vi "Wind_Turbine.vi"() -> (5 "Plug in titles":string[](array[string]), 7 "Plug in values":string[](array[string]))   [LabVIEW 2012]
uses:
  Globals/Meas_global.vi
  Globals/LDA_meas_global_1.vi
  <vilib>/Analysis/baseanly.llb/Mean (DBL).vi
  <vilib>/Analysis/NI_AALBase.lvlib
  <vilib>/Analysis/NI_AALPro.lvlib
panel:
  out "Blade 3 Every Pass":dbl[](graph)
  out "Blade 2 Every Pass":dbl[](graph)
  out "Blade 1 Every Pass":dbl[](graph)
  out "Blade Angles":dbl[][](graph)
  out "Blade Analysis":string[][](table)
  out "Blade Positions":dbl[][](graph)
  in  "Allow large changes?":bool
  out "Turbine RPMs":cluster{i32[], "All WTs":dbl[]}(graph)
  out "WT Numbers":string[](array[string])
  out "XY Graph":cluster{dbl[], dbl[]}[](graph)
  out "WT Revolution Start times":dbl[](array[numeric])
  out "Angle 3":dbl format="%#_3g"
  out "Angle 2":dbl format="%#_3g"
  out "Angle 1":dbl format="%#_3g"
  out "L Status Phase lock index":i32
  out "Laser Status Index":i32
  out "Laser Phase lock index":i32
  out "Laser Disp Index":i32
  out "Av Variance 3":dbl
  out "Av Variance 2":dbl
  out "Av Variance 1":dbl
  out "slope 3":dbl format="%#_3g"
  out "slope 2":dbl format="%#_3g"
  out "Mean Blade 3":cluster{dbl, "Angular Step":dbl, dbl[]}(graph)
  out "Mean Blade 2":cluster{dbl, "Angular Step":dbl, dbl[]}(graph)
  out "Av Disp 3":dbl
  out "Av Disp 2":dbl
  out "Av Disp 1":dbl
  out "slope 1":dbl format="%#_3g"
  in  "End Cut Deg":dbl
  in  "Start Cut Deg":dbl
  out "Mean Blade 1":cluster{dbl, "Angular Step":dbl, dbl[]}(graph)
  in  "Angular Step":dbl=1.0
  in  "Turbine to Phase Lock to":u16(ring) items=["RV (WT1)"]
  in  "Change Dem Voltages?":bool=TRUE
  out "All WTs":dbl[][](array[numeric]) format="%#.2g"
  out "WT trace index":dbl[][](array[numeric])
  in  "precision":string
  in  "Add Phase data to results file":bool
  in  "Separation Character":string="\t"
  in  "Output Directory":path
  in  "Save Phase averaged Profiles":bool
  out "Pulses per Rev":i32
  in  "Channel to Phase lock":i32[](listbox)
  # "Mean RPM      SD RPM           Max-Min"
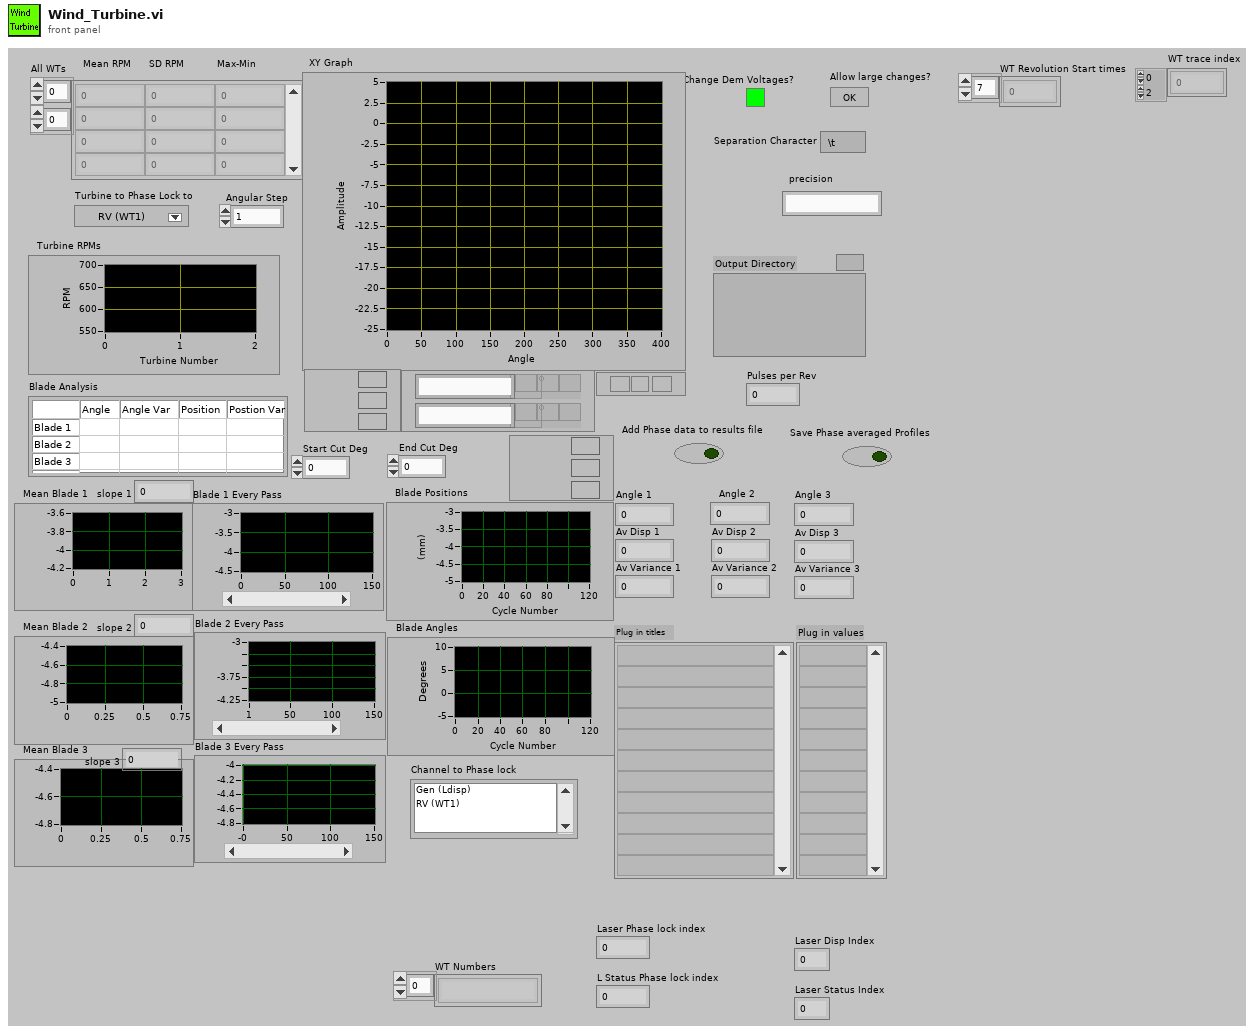
[diagram p1: front panel]
types:
  T1 = typedef "Post_Process.ctl" = enum16{"Take New Data", "Post Process Raw Data File"}
  T2 = typedef "Analysis_info_cluster.ctl" = cluster{"Colour":u32, "Inst type":T3, "Inst name":string, "Symbol":string, "Code name":string, "Extra Info":string, "Inst Array":T4, "Extra Titles":string[], "Extra Values":string[], "U":dbl, "u^2":dbl, "u^3":dbl, "u^4":dbl, "Skew_u":dbl, "Kurt_u":dbl, "Sd Error in Mean":dbl, "% u'/U":dbl, "X":dbl, "Y":dbl, "Z":dbl, "Timescale integral to 25%":dbl, "Sd Error in Variance":dbl, "Calib File":path, "Calib Constants":dbl[], "Output Position":bool, "Full Stats":bool, "Av Sampling Rate":dbl, "Av No of Samples":dbl, "Total Meas Time (s)":dbl, "ADAM Ch Name":string}
  T3 = typedef "Inst_type.ctl" = enum16{"Propeller anemometer", "Raw voltage", "Pressure Transducer", "Pitot-static tube", "Preston tube", "Hot wire", "Cross wire 1", "Cross wire 2", "Generic Linear", "Generic Polynomial", "Generic BackPoly", "Fast FID", "Thermocouple", "Cold wire", "Pulsed Wire", "LDA Vel", "LDA Tran time", "LDA Arr time"}
  T4 = typedef "Instrument_Array.ctl" = enum16{"PWA", "LDA", "Analogue"}
  T5 = typedef "Time_Trace_Cluster.ctl" = cluster{"Weighting":dbl[], "Time (s)":dbl[], "Voltage":dbl[], "Eng Values":dbl[]}
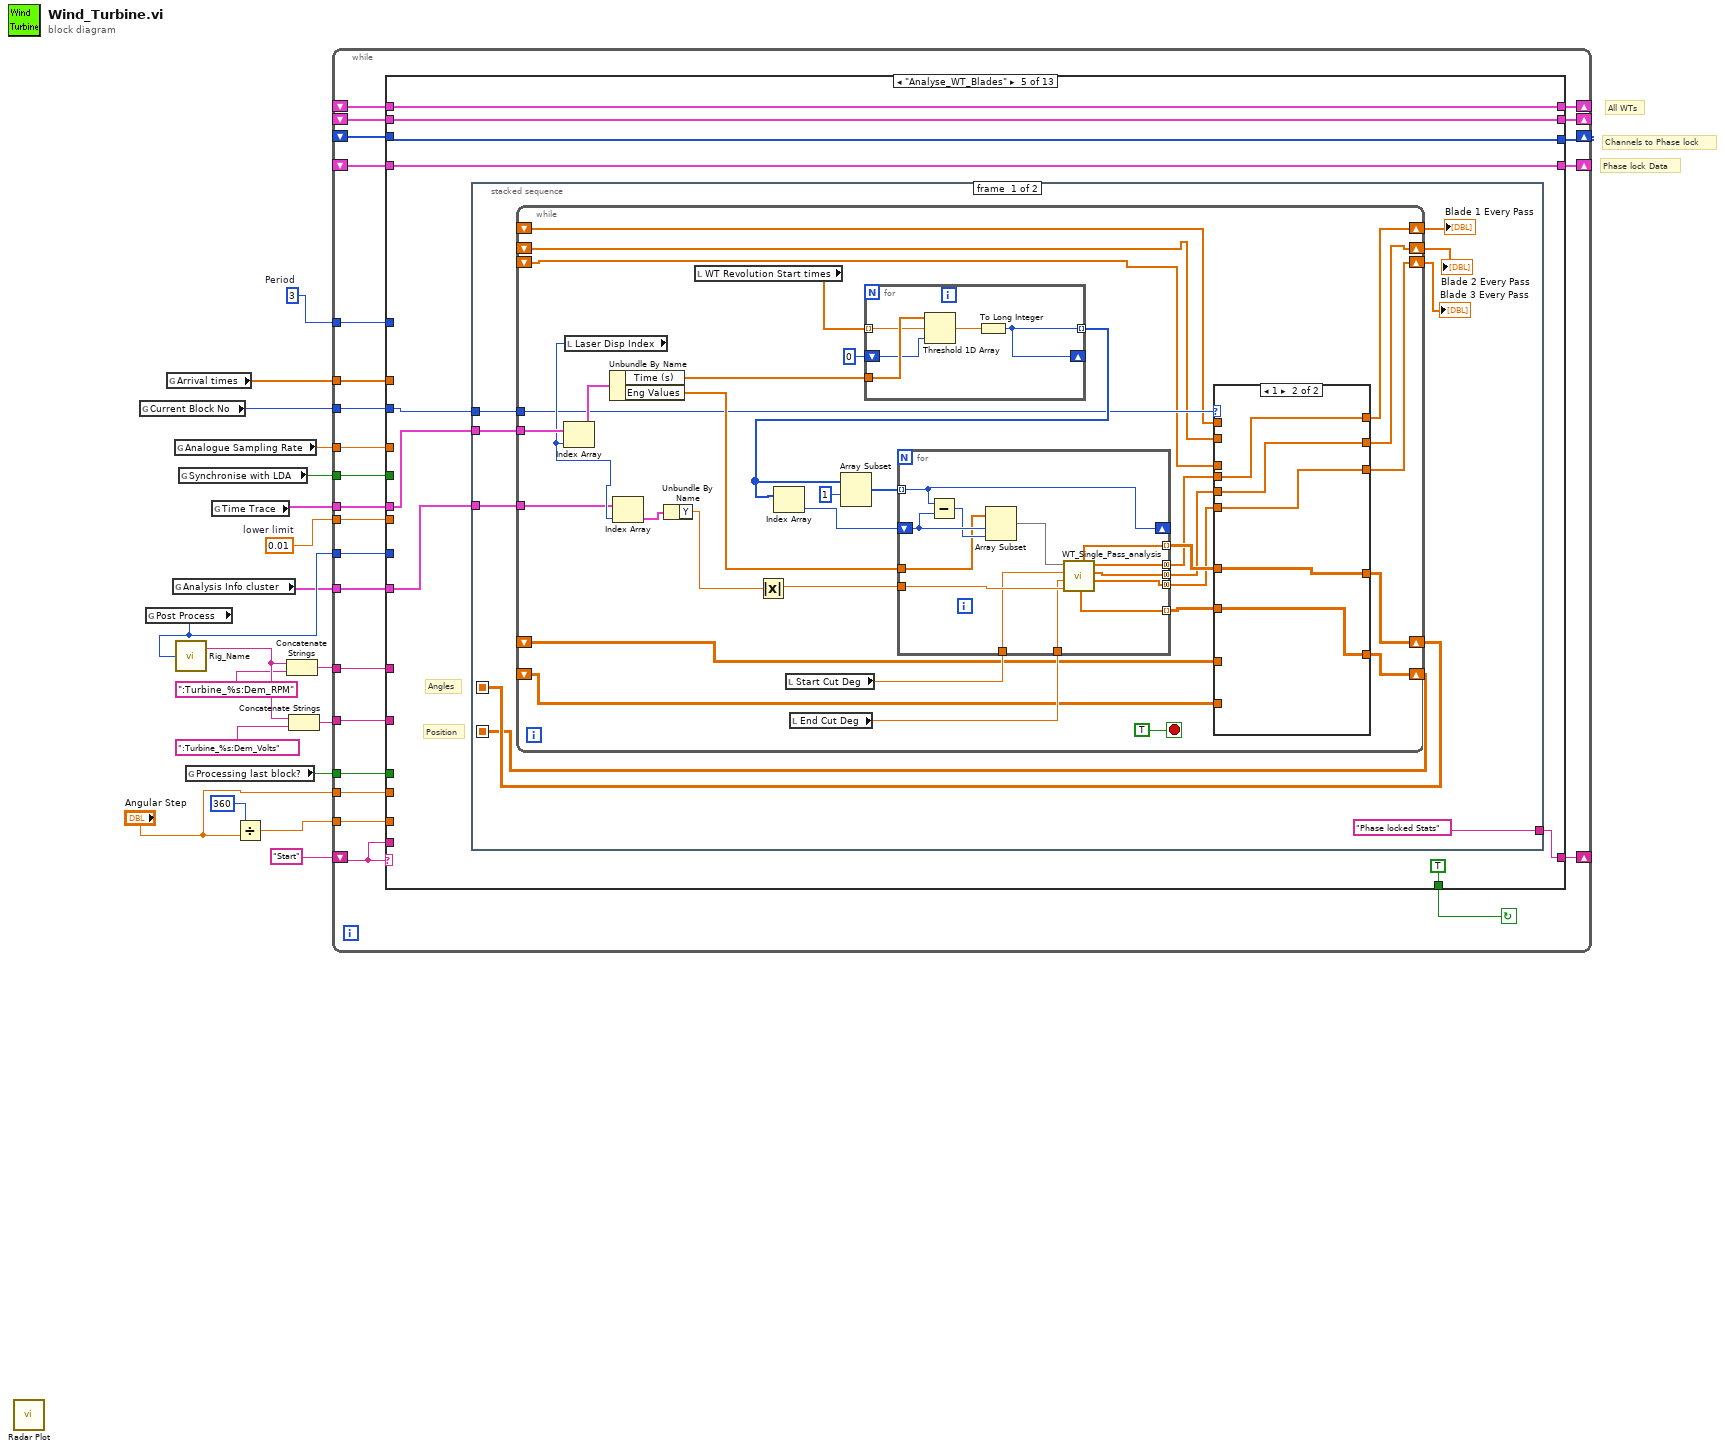
[diagram p0: block diagram]
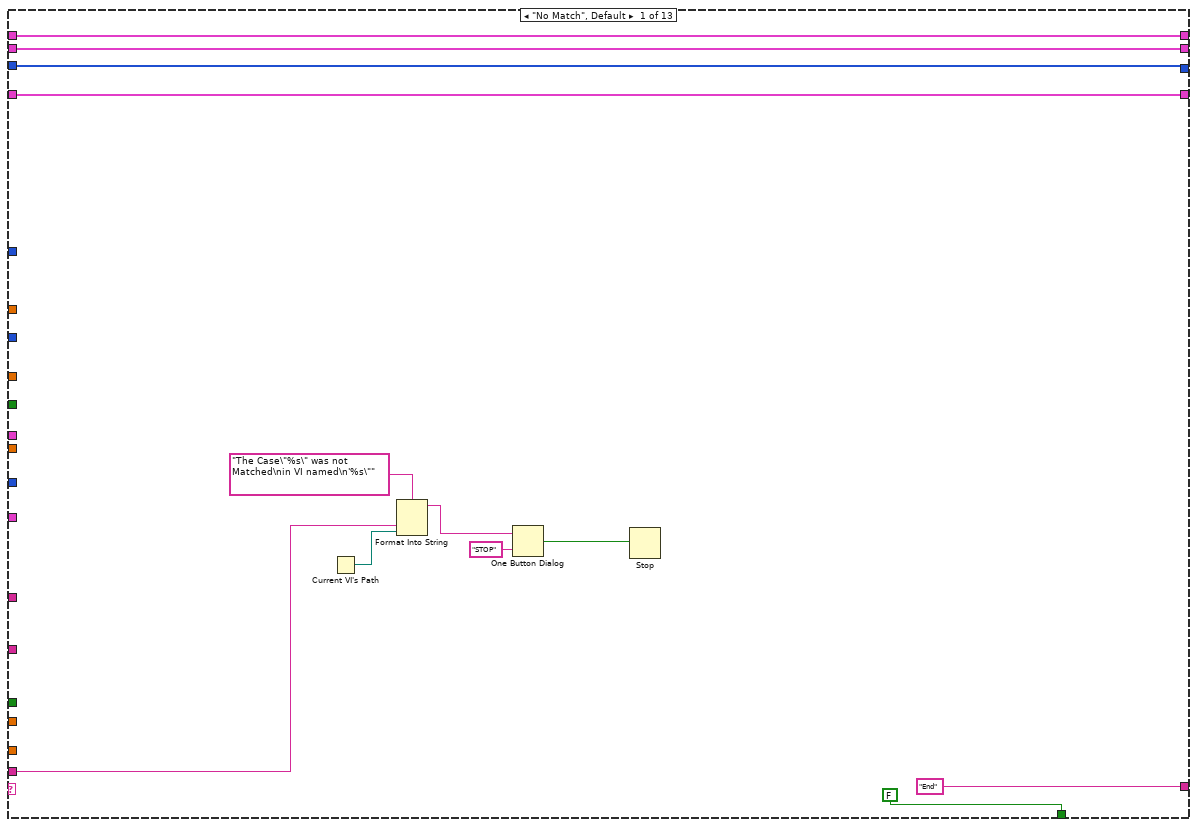
[diagram p2: hidden frame]
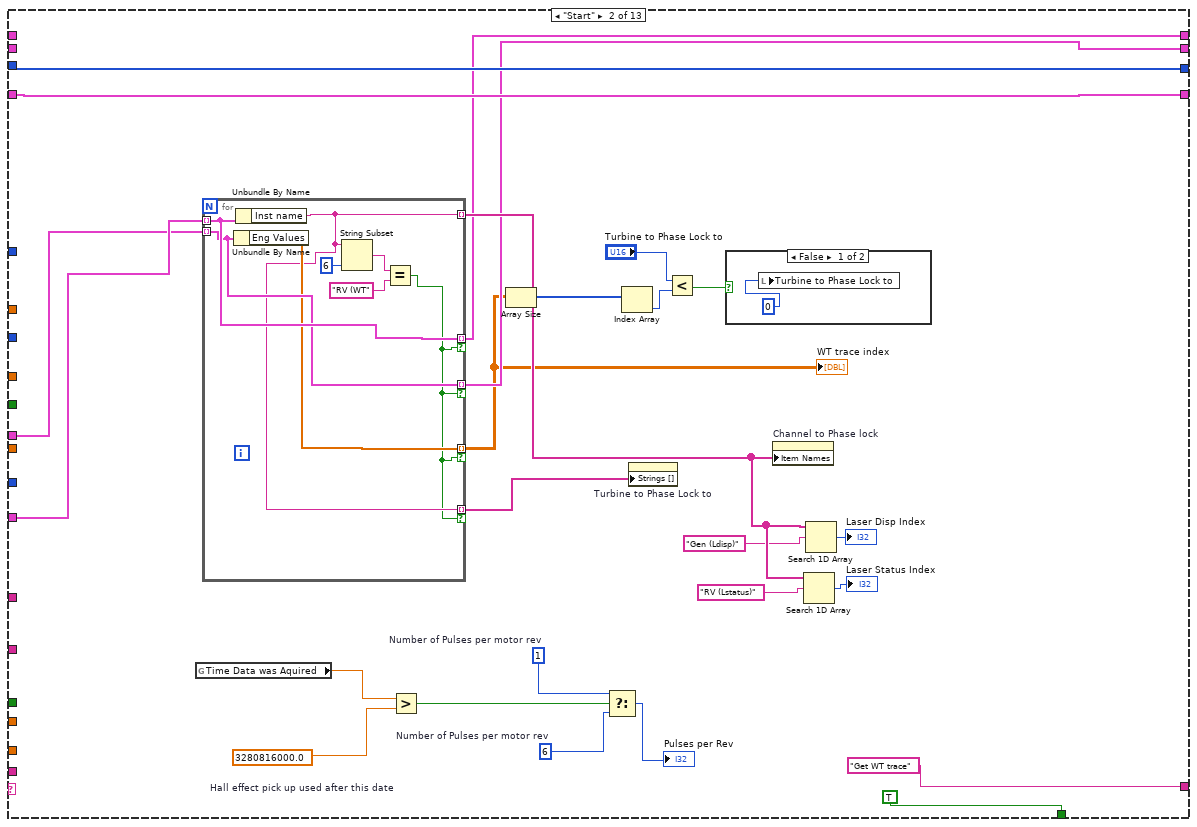
[diagram p3: hidden frame]
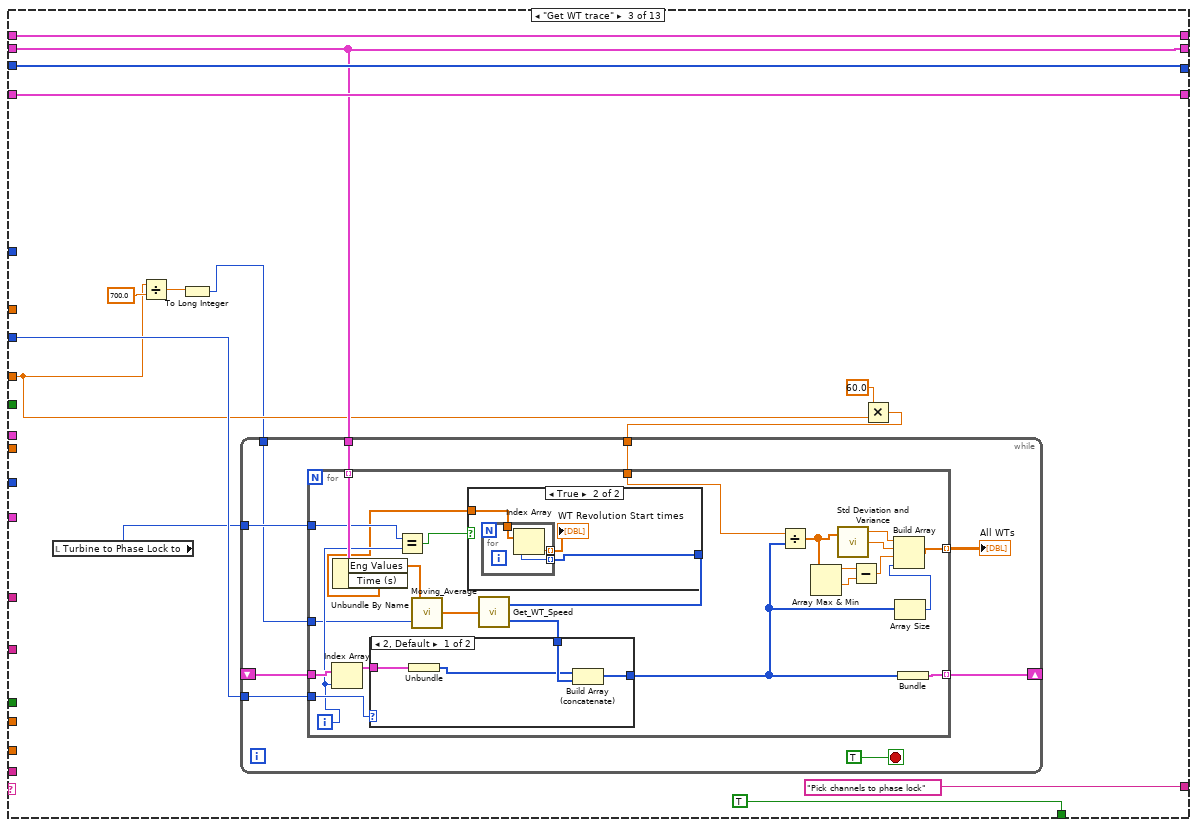
[diagram p5: hidden frame]
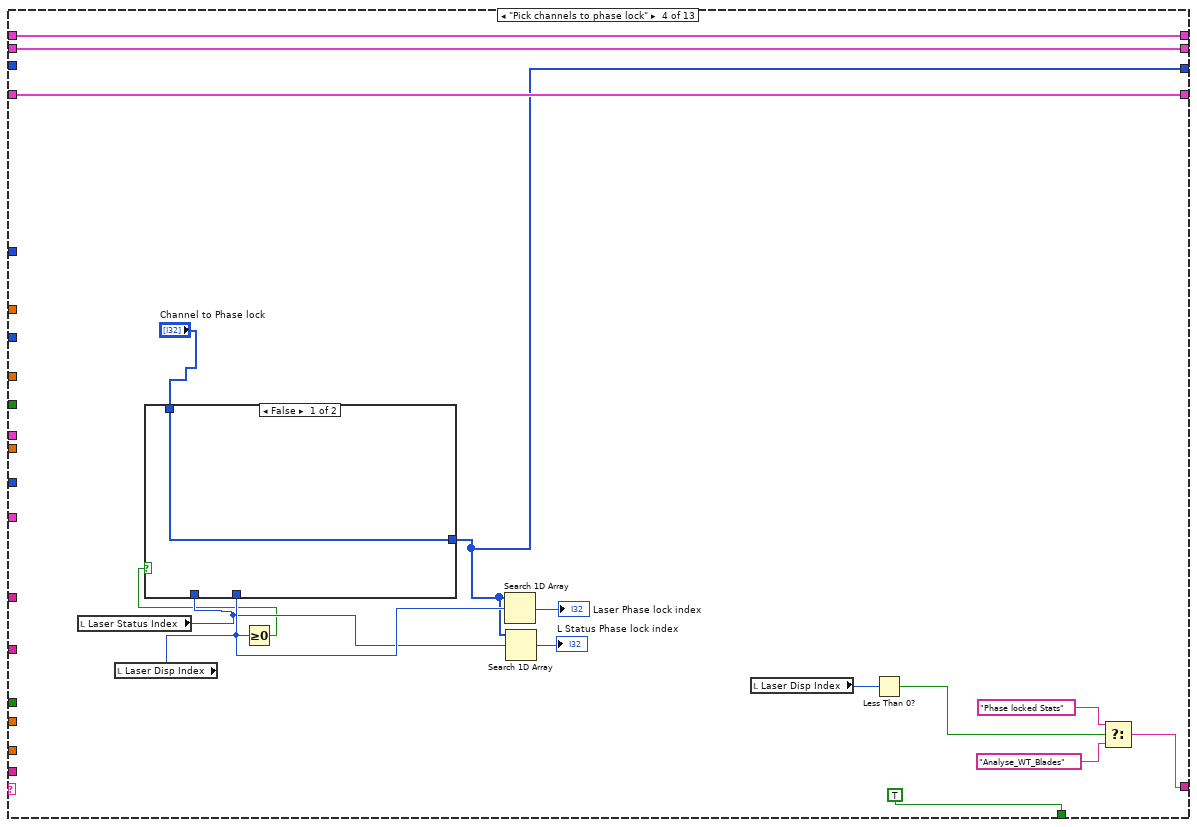
[diagram p8: hidden frame]
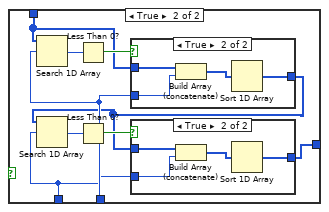
[diagram p9: hidden frame]
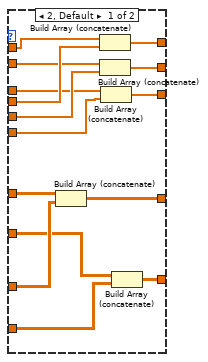
[diagram p12: hidden frame]
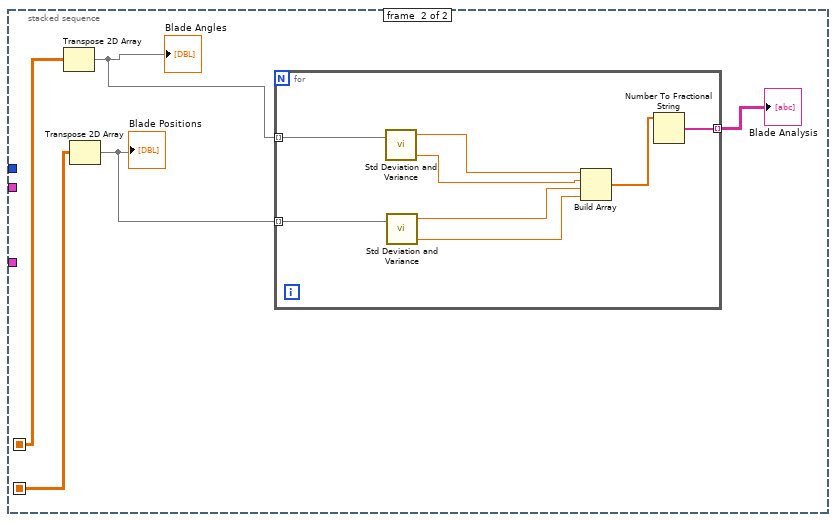
[diagram p13: hidden frame]
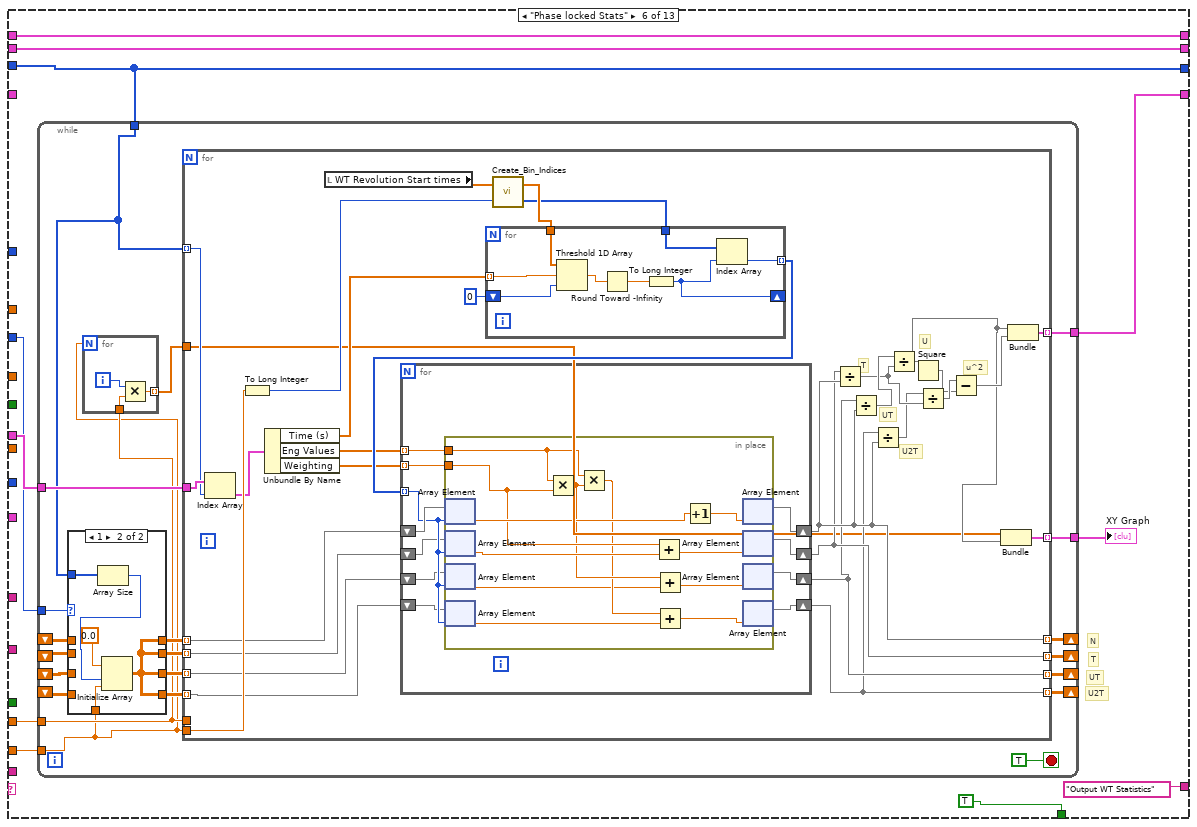
[diagram p14: hidden frame]
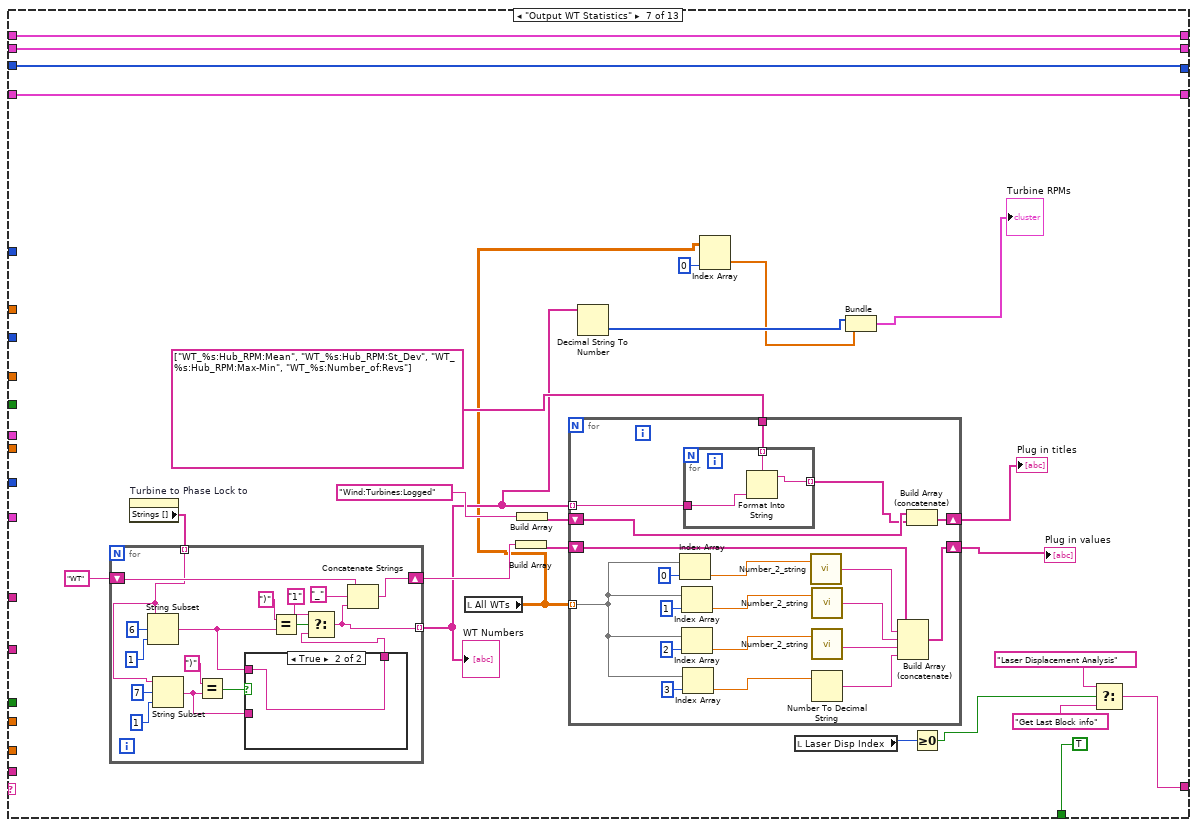
[diagram p16: hidden frame]
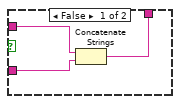
[diagram p17: hidden frame]
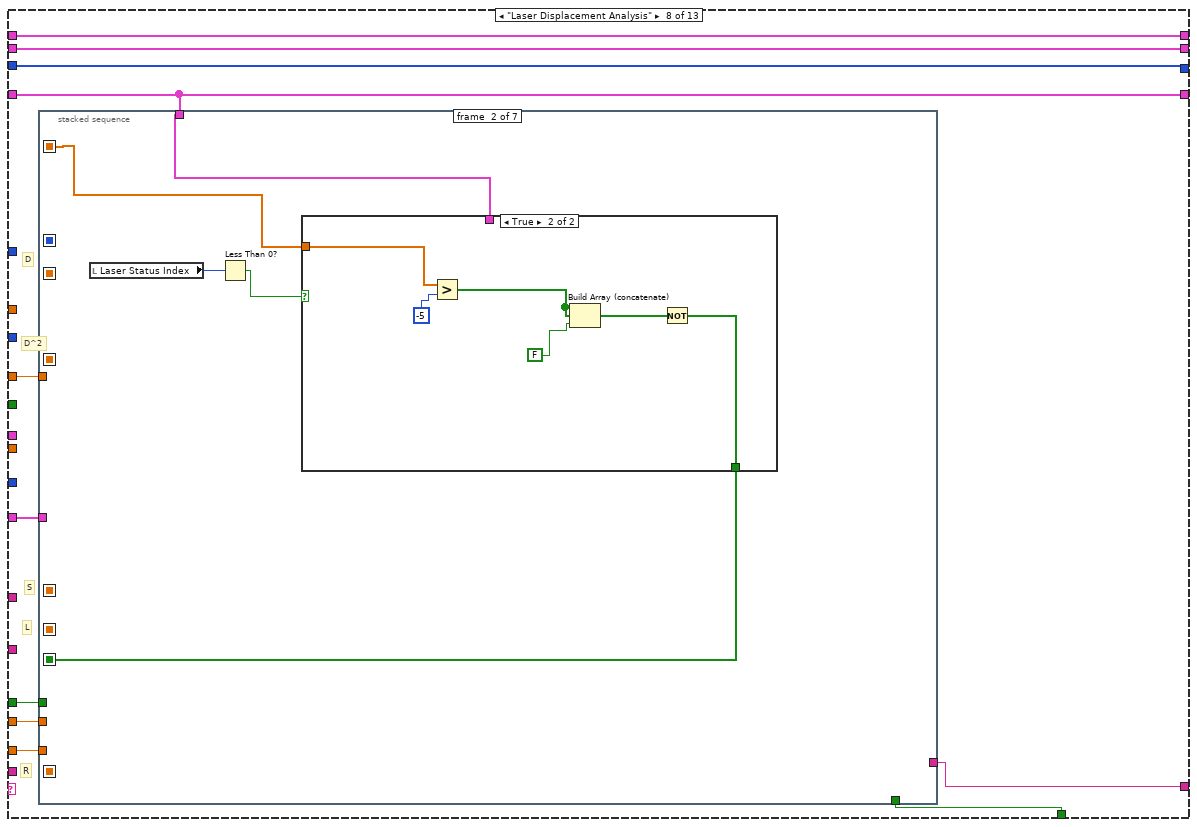
[diagram p18: hidden frame]
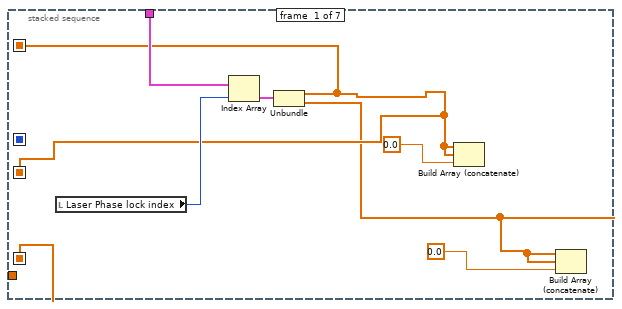
[diagram p19: hidden frame]
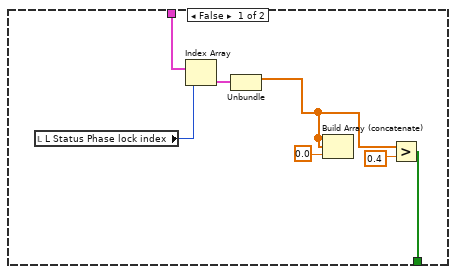
[diagram p20: hidden frame]
diagram:
  w17 = 3  # Period
  w18 = 0.01  # lower limit
  # "Phase lock Data"
  # "Channels to Phase lock"
  # "All WTs"
  n1 = call <vilib>:"Radar Plot.vi"() -> ()  [unwired: 15 in, 1 out]
  n2 = global read "Meas_global.vi" "Current Block No"() -> (w4:i32)
  n3 = global read "Meas_global.vi" "Post Process"() -> (w16:T1)
  n4 = global read "LDA_meas_global_1.vi" "Arrival times"() -> (w7:dbl[])
  n5 = global read "Meas_global.vi" "Analysis Info cluster"() -> (w6:T2[])
  n6 = global read "Meas_global.vi" "Analogue Sampling Rate"() -> (w19:dbl)
  n7 = call "Rig_Name.vi"("Post Process"=w16) -> ("Rig Setup before dash"=w13:string)  [unwired: 1 out]
  n8 = global read "Meas_global.vi" "Synchronise with LDA"() -> (w11:bool)
  n9 = global read "Meas_global.vi" "Processing last block?"() -> (w9:bool)
  n10 = global read "Meas_global.vi" "Time Trace"() -> (w2:T5[])
  n11 = Divide(x=360, y="Angular Step") -> (x/y=w5:dbl)
  n12 = Concatenate Strings(w13, ":Turbine_%s:Dem_RPM") -> (w12:string)
  n13 = Concatenate Strings(w13, ":Turbine_%s:Dem_Volts") -> (w15:string)
  n14 = while {
    tunnel: w4 -> [w44]
    tunnel: w19 -> [w43]
    tunnel: w15 -> [w42]
    tunnel: w12 -> [w41]
    tunnel: w18 -> [w40]
    tunnel: w17 -> [w39]
    tunnel: w16 -> [w38]
    tunnel: w11 -> [w37]
    tunnel: w6 -> [w36]
    shift-right: [w20] -> _
    shift-left: "Start" -> [w34]
    tunnel: w9 -> [w33]
    tunnel: w5 -> [w32]
    tunnel: w7 -> [w31]
    tunnel: "Angular Step" -> [w30]
    shift-right: [w29] -> _
    shift-left: _ -> [w28]
    shift-right: [w26] -> _
    shift-left: _ -> [w27]
    shift-right: [w25] -> _
    shift-left: _ -> [w24]
    tunnel: w2 -> [w23]
    shift-right: [w22] -> _
    shift-left: _ -> [w21]
    stop <- w35 continue-if-true
    n15 = case shown="\"Analyse_WT_Blades\"" w34 {
      tunnel: w44 -> [_ _ w100 _ w186 w291 _ _ _ _ _ _ _]
      tunnel: w43 -> [_ _ w93 _ _ _ _ w473 _ _ _ _ w857]
      tunnel: w42 -> [_ _ _ _ _ _ _ _ _ w747 _ _ _]
      tunnel: w41 -> [_ _ _ _ _ _ _ _ _ w722 _ _ _]
      tunnel: w40 -> [_ _ _ _ _ _ _ _ _ _ _ _ _]
      tunnel: w39 -> [_ _ _ _ _ _ _ _ _ _ _ _ _]
      tunnel: w38 -> [_ _ _ _ _ _ _ _ w707 _ _ _ _]
      tunnel: w37 -> [_ _ _ _ _ _ _ _ _ _ _ _ _]
      tunnel: w36 -> [_ w75 _ _ w188 _ _ w463 _ _ _ _ _]
      tunnel: ["End" "Get WT trace" "Pick channels to phase lock" w149 w185 "Output WT Statistics" w412 w468 w706 "End" ("f") "Check Folder Name" "Save Phase locked data" "End"] -> w20
      tunnel: [FALSE ("Change Control Voltage?") TRUE ("Processing last block?") TRUE TRUE ("Change Control Voltage?") TRUE ("Change Control Voltage?") TRUE TRUE ("Change Control Voltage?") w469 w705 FALSE ("Change Control Voltage?") w783 w834 FALSE ("Change Control Voltage?")] -> w35
      tunnel: w34 -> [w51 _ _ _ _ _ _ _ _ _ _ _ _]
      tunnel: w33 -> [_ _ _ _ _ _ _ w470 w704 _ w781 _ _]
      tunnel: w32 -> [_ _ _ _ _ w298 _ w472 _ _ w779 _ _]
      tunnel: w31 -> [_ _ _ _ _ _ _ _ _ _ _ _ _]
      tunnel: w30 -> [_ _ _ _ _ w297 _ w471 _ _ _ _ w851]
      tunnel: [w48 w60 w96 w164 w193 w296 w409 w467 w703 w721 w778 w832 w854] -> w29
      tunnel: w28 -> [w48 _ w96 w164 w193 w296 w409 w467 w703 w721 w778 w832 w854]
      tunnel: w27 -> [w47 w61 w98 _ w191 w292 w408 w466 w702 w720 w777 w831 w853]
      tunnel: [w47 w61 w98 w155 w191 w292 w408 w466 w702 w720 w777 w831 w853] -> w26
      tunnel: [w46 w62 w97 w159 w190 w290 w407 w464 w701 w719 w775 w830 w852] -> w25
      tunnel: w24 -> [w46 w62 w97 w159 w190 _ w407 w464 w701 w719 w775 w830 w852]
      tunnel: w23 -> [_ w63 _ _ w189 w293 _ _ _ _ _ _ _]
      tunnel: [w45 w59 w95 w158 w192 w294 w406 w465 w700 w718 w776 w829 w850] -> w22
      tunnel: w21 -> [w45 _ w95 w158 w192 w294 w406 w465 w700 w718 w776 w829 w850]
      frame "No Match", Default {
        n16 = Current VI's Path() -> (path=w52:path)
        n17 = Format Into String(format string="The Case\"%s\" was not Matched\nin VI named\n'%s\"" ("Format String"), w51, w52) -> (resulting string=w55:string)  [unwired: 2 in, 1 out]
        n18 = One Button Dialog(message=w55, button name ("OK")="STOP") -> (true=w53:bool)
        n19 = Stop(stop? (T)=w53) -> ()
      }
      frame "Start" {
        w76 = 6  # Number of Pulses per motor rev
        w77 = 1  # Number of Pulses per motor rev
        w79 = 3280816000.0  # Hall effect pick up used after this date
        n20 = global read "Meas_global.vi" "Time Data was Aquired"() -> (w80:dbl)
        n21 = for {
          tunnel: w75 -> [w87] mode=indexing
          tunnel: [w84] -> w68 mode=indexing
          tunnel: w63 -> [w86] mode=indexing
          tunnel: [w87] -> w60 mode=indexing if=w83
          tunnel: [w86] -> w59 mode=indexing if=w83
          tunnel: [w85] -> w58 mode=indexing if=w83
          tunnel: [w84] -> w57 mode=indexing if=w83
          n22 = Unbundle By Name(w86) -> ("Eng Values"=w85:dbl[])
          n23 = Unbundle By Name(w87) -> ("Inst name"=w84:string)
          n24 = String Subset(string=w84, length (rest)=6 ("length (rest)")) -> (substring=w88:string)  [unwired: 1 out]
          n25 = Equal?(x=w88, y="RV (WT") -> (x = y?=w83:bool)
        }
        "WT trace index" <- w58
        n26 = Greater?(x=w80, y=w79) -> (0:w78:bool)
        n27 = Array Size(array=w58) -> (size(s)=w65:i32[])
        n28 = Select(t=w77, s=w78, f=w76) -> (s? t:f=→"Pulses per Rev":i32)
        n29 = Index Array(array=w65) -> (element=w64:i32)  [unwired: 1 in]
        n30 = property on="Turbine to Phase Lock to" class="Ring (strict)"("Strings []"=w57) -> ()  [unwired: 2 in, 2 out]
        n31 = Less?(x="Turbine to Phase Lock to", y=w64) -> (x < y?=w71:bool)
        n32 = case shown="False" w71 {
          frame False {
            n33 = local write "Turbine to Phase Lock to"(0) -> ()
          }
          frame True {
          }
        }
        n34 = property on="Channel to Phase lock" class="LstBox (strict)"("Item Names"=w68) -> ()  [unwired: 2 in, 2 out]
        n35 = Search 1D Array(1D array=w68, element="RV (Lstatus)") -> (index of element=→"Laser Status Index":i32)  [unwired: 1 in]
        n36 = Search 1D Array(1D array=w68, element="Gen (Ldisp)") -> (index of element=→"Laser Disp Index":i32)  [unwired: 1 in]
      }
      frame "Get WT trace" {
        n37 = local read "Turbine to Phase Lock to"() -> (w99:u16)
        n38 = Divide(x=w93, y=700.0) -> (x/y=w92:dbl)
        n39 = To Long Integer(number=w92) -> (32bit integer=w91:i32)
        n40 = Multiply(x=60.0, y=w93) -> (x*y=w101:dbl)
        n41 = while {
          tunnel: w100 -> [w113]
          shift-right: [w108] -> _
          shift-left: _ -> [w112]
          tunnel: w101 -> [w111]
          tunnel: w95 -> [w107]
          tunnel: w99 -> [w106]
          tunnel: w91 -> [w105]
          stop <- TRUE stop-if-true
          n42 = for {
            tunnel: w113 -> [w136]
            tunnel: w112 -> [w126]
            tunnel: w111 -> [w134]
            tunnel: [w127] -> w109 mode=indexing
            tunnel: [w122] -> w108 mode=indexing
            tunnel: w107 -> [w121] mode=indexing
            tunnel: w106 -> [w117]
            tunnel: w105 -> [w114]
            i -> [w118]
            n43 = Index Array(array=w126, index=w118) -> (element=w125:cluster{"Samples per pulse":i32[]})
            n44 = Unbundle By Name(w121) -> ("Eng Values"=w120:dbl[], "Time (s)"=w115:dbl[])
            n45 = Equal?(x=w117, y=w118) -> (x = y?=w116:bool)
            n46 = call "Moving_Average.vi"("Period"=w114, "Input Array"=w120) -> ("N+1-Period"=w137:dbl[])
            n47 = call "Get_WT_Speed.vi"("Opto Trace"=w137) -> ("Start Cycle Index"=w119:i32[], "Samples per pulse"=w135:i32[])
            n48 = case shown="2, Default" w136 {
              tunnel: [w146 w148] -> w123
              tunnel: w135 -> [w147 w148]
              tunnel: w125 -> [w145 _]
              frame 2, Default {
                n49 = Unbundle(w145) -> ("Samples per pulse"=w144:i32[])
                n50 = Build Array (concatenate)(w144, w147) -> (w146:i32[])
              }
              frame 1 {
              }
            }
            n51 = case shown="True" w116 {
              tunnel: w119 -> [_ w140]
              tunnel: w115 -> [_ w139]
              frame False {
              }
              frame True {
                n52 = for {
                  tunnel: w140 -> [w143] mode=indexing
                  tunnel: w139 -> [w142]
                  tunnel: [w141] -> w138 mode=indexing
                  n53 = Index Array(array=w142, index=w143) -> (element=w141:dbl)
                }
                "WT Revolution Start times" <- w138
              }
            }
            n54 = Divide(x=w134, y=w123) -> (x/y=w131:dbl[])
            n55 = Array Max & Min(array=w131) -> (max value=w133:dbl, min value=w132:dbl)  [unwired: 2 out]
            n56 = call <vilib>:"Std Deviation and Variance.vi"("X"=w131) -> ("mean"=w130:dbl, "standard deviation"=w129:dbl)  [unwired: 1 in, 1 out]
            n57 = Subtract(x=w133, y=w132) -> (x-y=w128:dbl)
            n58 = Array Size(array=w123) -> (size(s)=w124:i32)
            n59 = Build Array(w130, w129, w128, w124) -> (w127:dbl[])
            n60 = Bundle("Samples per pulse"=w123) -> (w122:cluster{"Samples per pulse":i32[]})  [unwired: 1 in]
          }
          "All WTs" <- w109
        }
      }
      frame "Pick channels to phase lock" {
        n61 = local read "Laser Status Index"() -> (w161:i32)
        n62 = local read "Laser Disp Index"() -> (w162:i32)
        n63 = Greater Or Equal To 0?(x=w162) -> (x >= 0?=w160:bool)
        n64 = case shown="False" w160 {
          tunnel: "Channel to Phase lock" -> [w165 w172]
          tunnel: w162 -> [_ w171]
          tunnel: [w165 w168] -> w155
          tunnel: w161 -> [_ w166]
          frame False {
          }
          frame True {
            n65 = Search 1D Array(1D array=w172, element=w171) -> (index of element=w174:i32)  [unwired: 1 in]
            n66 = Less Than 0?(x=w174) -> (x < 0?=w173:bool)
            n67 = case shown="True" w173 {
              tunnel: w172 -> [w180 w184]
              tunnel: w171 -> [_ w183]
              tunnel: [w180 w181] -> w167
              frame False {
              }
              frame True {
                n68 = Build Array (concatenate)(w184, w183) -> (w182:i32[])
                n69 = Sort 1D Array(array=w182) -> (sorted array=w181:i32[])
              }
            }
            n70 = Search 1D Array(1D array=w167, element=w166) -> (index of element=w169:i32)  [unwired: 1 in]
            n71 = Less Than 0?(x=w169) -> (x < 0?=w170:bool)
            n72 = case shown="True" w170 {
              tunnel: w167 -> [w175 w179]
              tunnel: w166 -> [_ w178]
              tunnel: [w175 w176] -> w168
              frame False {
              }
              frame True {
                n73 = Build Array (concatenate)(w179, w178) -> (w177:i32[])
                n74 = Sort 1D Array(array=w177) -> (sorted array=w176:i32[])
              }
            }
          }
        }
        n75 = Search 1D Array(1D array=w155, element=w162) -> (index of element=→"Laser Phase lock index":i32)  [unwired: 1 in]
        n76 = Search 1D Array(1D array=w155, element=w161) -> (index of element=→"L Status Phase lock index":i32)  [unwired: 1 in]
        n77 = local read "Laser Disp Index"() -> (w153:i32)
        n78 = Less Than 0?(x=w153) -> (x < 0?=w152:bool)
        n79 = Select(t="Phase locked Stats" ("f"), s=w152, f="Analyse_WT_Blades") -> (s? t:f=w149:string)
      }
      frame "Analyse_WT_Blades" {
        # "Position"
        # "Angles"
        n80 = stacked-sequence {
          seq-local: [w197 _] -> [_ w278]
          seq-local: [w198 _] -> [_ w279]
          tunnel: w189 -> [w202 _]
          tunnel: w188 -> [w201 _]
          tunnel: w186 -> [w200 _]
          tunnel: ["Phase locked Stats" ("f") _] -> w185
          frame #0 {
            n81 = while {
              tunnel: w202 -> [w236]
              tunnel: w201 -> [w225]
              shift-right: [w215] -> w198
              shift-left: _ -> [w216]
              shift-right: [w212] -> w197
              shift-left: _ -> [w213]
              tunnel: w200 -> [w218]
              shift-right: [w210] -> w196
              shift-left: _ -> [w209]
              shift-right: [w205] -> w195
              shift-left: _ -> [w206]
              shift-right: [w203] -> w194
              shift-left: _ -> [w204]
              stop <- TRUE stop-if-true
              n82 = local read "Laser Disp Index"() -> (w226:i32)
              n83 = Index Array(array=w236, index=w226) -> (element=w235:T5)
              n84 = Unbundle By Name(w235) -> ("Time (s)"=w234:dbl[], "Eng Values"=w227:dbl[])
              n85 = Index Array(array=w225, index=w226) -> (element=w224:T2)
              n86 = Unbundle By Name(w224) -> ("Y"=w223:dbl)
              n87 = local read "WT Revolution Start times"() -> (w233:dbl[])
              n88 = Absolute Value(x=w223) -> (abs(x)=w222:dbl)
              n89 = local read "Start Cut Deg"() -> (w221:dbl)
              n90 = local read "End Cut Deg"() -> (w220:dbl)
              n91 = for {
                tunnel: w234 -> [w274]
                tunnel: w233 -> [w273] mode=indexing
                shift-right: [w270] -> _
                shift-left: 0 -> [w272]
                tunnel: [w270] -> w230 mode=indexing
                n92 = Threshold 1D Array(1:w272, 2:w273, 3:w274) -> (0:w271:dbl)
                n93 = To Long Integer(number=w271) -> (32bit integer=w270:i32)
              }
              n94 = Index Array(array=w230) -> (element=w229:i32)  [unwired: 1 in]
              n95 = Array Subset(array=w230, index=1) -> (w228:i32[])  [unwired: 1 in]
              n96 = for {
                shift-right: [w268] -> _
                shift-left: w229 -> [w269]
                tunnel: w228 -> [w268] mode=indexing
                tunnel: w227 -> [w266]
                tunnel: w222 -> [w264]
                tunnel: [w260] -> w217 mode=indexing
                tunnel: [w263] -> w214 mode=indexing
                tunnel: w221 -> [w262]
                tunnel: w220 -> [w261]
                tunnel: [w259] -> w211 mode=concatenating
                tunnel: [w258] -> w208 mode=concatenating
                tunnel: [w257] -> w207 mode=concatenating
                n97 = Subtract(x=w268, y=w269) -> (x-y=w267:i32)
                n98 = Array Subset(array=w266, index=w269, length=w267) -> (w265:dbl[])
                n99 = call "WT_Single_Pass_analysis.vi"("Displacement"=w265, "Start Cut Deg"=w262, "End Cut Deg"=w261, "Radius"=w264) -> ("Blade Angles"=w260:dbl[], "Blade Positions"=w263:dbl[], "Blade1"=w259:dbl[], "Blade 2"=w258:dbl[], "Blade 3"=w257:dbl[])  [unwired: 1 in]
              }
              n100 = case shown="1" w218 {
                tunnel: w217 -> [w251 w256]
                tunnel: w216 -> [w250 _]
                tunnel: [w249 w256] -> w215
                tunnel: w214 -> [w248 w255]
                tunnel: w213 -> [w247 _]
                tunnel: [w246 w255] -> w212
                tunnel: w211 -> [w245 w254]
                tunnel: [w243 w254] -> w210
                tunnel: w209 -> [w244 _]
                tunnel: w208 -> [w242 w253]
                tunnel: w207 -> [w241 w252]
                tunnel: w206 -> [w240 _]
                tunnel: [w239 w253] -> w205
                tunnel: w204 -> [w238 _]
                tunnel: [w237 w252] -> w203
                frame 2, Default {
                  n101 = Build Array (concatenate)(w251, w250) -> (w249:dbl[][])
                  n102 = Build Array (concatenate)(w244, w245) -> (w243:dbl[])
                  n103 = Build Array (concatenate)(w240, w242) -> (w239:dbl[])
                  n104 = Build Array (concatenate)(w238, w241) -> (w237:dbl[])
                  n105 = Build Array (concatenate)(w248, w247) -> (w246:dbl[][])
                }
                frame 1 {
                }
              }
            }
            "Blade 1 Every Pass" <- w196
            "Blade 3 Every Pass" <- w194
            "Blade 2 Every Pass" <- w195
          }
          frame #1 {
            n106 = Transpose 2D Array(2D array=w279) -> (transposed array=w276:dbl[][])
            "Blade Angles" <- w276
            n107 = Transpose 2D Array(2D array=w278) -> (transposed array=w277:dbl[][])
            "Blade Positions" <- w277
            n108 = for {
              tunnel: w276 -> [w287] mode=indexing
              tunnel: w277 -> [w286] mode=indexing
              tunnel: [w280] -> w275 mode=indexing
              n109 = call <vilib>:"Std Deviation and Variance.vi"("X"=w287) -> ("mean"=w285:dbl, "variance"=w284:dbl)  [unwired: 1 in, 1 out]
              n110 = call <vilib>:"Std Deviation and Variance.vi"("X"=w286) -> ("mean"=w283:dbl, "variance"=w282:dbl)  [unwired: 1 in, 1 out]
              n111 = Build Array(w285, w284, w283, w282) -> (w281:dbl[])
              n112 = Number To Fractional String(number=w281) -> (F-format string=w280:string[])  [unwired: 3 in]
            }
            "Blade Analysis" <- w275
          }
        }
      }
      frame "Phase locked Stats" {
        # "N"
        # "U2T"
        # "UT"
        # "T"
        n113 = while {
          tunnel: w298 -> [w299]
          tunnel: w297 -> [w301]
          tunnel: w292 -> [w316]
          shift-right: [w305] -> _
          shift-left: _ -> [w311]
          tunnel: w293 -> [w318]
          shift-right: [w304] -> _
          shift-left: _ -> [w310]
          shift-right: [w303] -> _
          shift-left: _ -> [w309]
          shift-right: [w302] -> _
          shift-left: _ -> [w308]
          tunnel: w291 -> [w317]
          tunnel: [w307] -> w290
          tunnel: [w306] -> w289
          stop <- TRUE stop-if-true
          n114 = case shown="1" w317 {
            tunnel: w299 -> [_ w330]
            tunnel: w316 -> [_ w329]
            tunnel: [w326 w327] -> w315
            tunnel: [w325 w327] -> w314
            tunnel: [w324 w327] -> w313
            tunnel: [w323 w327] -> w312
            tunnel: w311 -> [w326 _]
            tunnel: w310 -> [w325 _]
            tunnel: w309 -> [w324 _]
            tunnel: w308 -> [w323 _]
            frame 2, Default {
            }
            frame 1 {
              n115 = Array Size(array=w329) -> (size(s)=w328:i32)
              n116 = Initialize Array(0.0, w328, w330) -> (w327:dbl[][])
            }
          }
          n117 = for {
            N: w299 -> [_]
            tunnel: w301 -> [w321]
            tunnel: [w320] -> w300 mode=indexing
            i -> [w322]
            n118 = Multiply(x=w322, y=w321) -> (x*y=w320:dbl)
          }
          n119 = for {
            tunnel: w299 -> [w357]
            tunnel: w301 -> [_]
            tunnel: w316 -> [w352] mode=indexing
            tunnel: w318 -> [w353]
            tunnel: w315 -> [w340] mode=indexing
            tunnel: [w336] -> w305 mode=indexing
            tunnel: [w335] -> w304 mode=indexing
            tunnel: [w334] -> w303 mode=indexing
            tunnel: [w333] -> w302 mode=indexing
            tunnel: w314 -> [w339] mode=indexing
            tunnel: w313 -> [w338] mode=indexing
            tunnel: w312 -> [w337] mode=indexing
            tunnel: [w343] -> w307 mode=indexing
            tunnel: [w341] -> w306 mode=indexing
            tunnel: w300 -> [w332]
            # "u^2"
            # "U"
            # "U2T"
            # "UT"
            # "T"
            n120 = Index Array(array=w353, index=w352) -> (element=w351:T5)
            n121 = To Long Integer(number=w357) -> (32bit integer=w356:i32)
            n122 = Unbundle By Name(w351) -> ("Time (s)"=w355:dbl[], "Eng Values"=w354:dbl[], "Weighting"=w350:dbl[])
            n123 = local read "WT Revolution Start times"() -> (w361:dbl[])
            n124 = call "Create_Bin_Indices.vi"("No Of Bins"=w356, "Cycle Start TIme"=w361) -> ("Bin Number"=w359:i32[], "Bin Start Time"=w360:dbl[])
            n125 = for {
              tunnel: w360 -> [w393]
              tunnel: w355 -> [w392] mode=indexing
              shift-right: [w389] -> _
              shift-left: 0 -> [w386]
              tunnel: w359 -> [w390]
              tunnel: [w388] -> w358 mode=indexing
              n126 = Threshold 1D Array(1:w386, 2:w392, 3:w393) -> (0:w391:dbl)
              n127 = Round Toward -Infinity(1:w391) -> (0:w387:dbl)
              n128 = To Long Integer(number=w387) -> (32bit integer=w389:i32)
              n129 = Index Array(array=w390, index=w389) -> (element=w388:i32)
            }
            n130 = for {
              tunnel: w358 -> [w372] mode=indexing
              tunnel: w354 -> [w364] mode=indexing
              tunnel: w350 -> [w363] mode=indexing
              shift-right: [w368] -> w336
              shift-left: w340 -> [w373]
              shift-right: [w367] -> w335
              shift-left: w339 -> [w369]
              shift-right: [w366] -> w334
              shift-left: w338 -> [w370]
              shift-right: [w365] -> w333
              shift-left: w337 -> [w371]
              n131 = in-place {
                in-place-border: w364 -> [w378]
                in-place-border: w363 -> [w381]
                n132 = in-place-array #1(w373, w372) -> (w385:dbl)
                n133 = in-place-array #2(w369, w372) -> (w383:dbl)
                n134 = in-place-array #3(w370, w372) -> (w375:dbl)
                n135 = in-place-array #4(w371, w372) -> (w374:dbl)
                n136 = Multiply(x=w378, y=w381) -> (x*y=w380:dbl)
                n137 = Multiply(x=w378, y=w380) -> (x*y=w379:dbl)
                n138 = Add(x=w381, y=w383) -> (x+y=w382:dbl)
                n139 = Add(x=w380, y=w375) -> (x+y=w376:dbl)
                n140 = Add(x=w379, y=w374) -> (x+y=w377:dbl)
                n141 = Increment(x=w385) -> (x+1=w384:dbl)
                n142 = in-place-array #1(w384) -> (w368:dbl[])  [unwired: 1 out]
                n143 = in-place-array #2(w382) -> (w367:dbl[])  [unwired: 1 out]
                n144 = in-place-array #3(w376) -> (w366:dbl[])  [unwired: 1 out]
                n145 = in-place-array #4(w377) -> (w365:dbl[])  [unwired: 1 out]
              }
            }
            n146 = Divide(x=w335, y=w336) -> (x/y=w348:dbl[])
            n147 = Divide(x=w334, y=w336) -> (x/y=w349:dbl[])
            n148 = Divide(x=w333, y=w336) -> (x/y=w347:dbl[])
            n149 = Divide(x=w349, y=w348) -> (x/y=w342:dbl[])
            n150 = Square(x=w342) -> (x^2=w345:dbl[])
            n151 = Divide(x=w347, y=w348) -> (x/y=w346:dbl[])
            n152 = Subtract(x=w346, y=w345) -> (x-y=w344:dbl[])
            n153 = Bundle(w332, w342) -> (w341:cluster{dbl[], dbl[]})  [unwired: 1 in]
            n154 = Bundle(w342, w344) -> (w343:cluster{dbl[], dbl[]})  [unwired: 1 in]
          }
        }
        "XY Graph" <- w289
      }
      frame "Output WT Statistics" {
        n155 = property on="Turbine to Phase Lock to" class="Ring (strict)"() -> ("Strings []"=w404:string[])  [unwired: 2 in, 2 out]
        n156 = for {
          shift-right: [w433] -> w401
          shift-left: "WT" -> [w434]
          tunnel: w404 -> [w424] mode=indexing
          tunnel: [w429] -> w399 mode=indexing
          n157 = String Subset(string=w424, offset (0)=6, length (rest)=1 ("length (rest)")) -> (substring=w420:string)
          n158 = String Subset(string=w424, offset (0)=7, length (rest)=1 ("length (rest)")) -> (substring=w419:string)
          n159 = Equal?(x=")", y=w419) -> (x = y?=w422:bool)
          n160 = case shown="True" w422 {
            tunnel: [w436 w439] -> w421
            tunnel: w420 -> [w438 w439]
            tunnel: w419 -> [w437 _]
            frame False {
              n161 = Concatenate Strings(w438, w437) -> (w436:string)
            }
            frame True {
            }
          }
          n162 = Equal?(x=")", y=w420) -> (x = y?=w430:bool)
          n163 = Select(t="1", s=w430, f=w421) -> (s? t:f=w429:string)
          n164 = Concatenate Strings(w434, "_", w429) -> (w433:string)
        }
        "WT Numbers" <- w399
        n165 = local read "All WTs"() -> (w398:dbl[][])
        n166 = Build Array(w401) -> (w400:string[])
        n167 = Build Array("Wind:Turbines:Logged") -> (w402:string[])
        n168 = for {
          tunnel: w398 -> [w451] mode=indexing
          shift-right: [w445] -> w418
          shift-left: w400 -> [w446]
          shift-right: [w441] -> w416
          shift-left: w402 -> [w443]
          tunnel: string[] ["WT_%s:Hub_RPM:Mean", "WT_%s:Hub_RPM:St_Dev", "WT_%s:Hub_RPM:Max-Min", "WT_%s:Number_of:Revs"] ("Plug in titles") -> [w444]
          tunnel: w399 -> [w440] mode=indexing
          n169 = Index Array(array=w451, index=0) -> (element=w450:dbl)
          n170 = Index Array(array=w451, index=1) -> (element=w449:dbl)
          n171 = Index Array(array=w451, index=2) -> (element=w448:dbl)
          n172 = Index Array(array=w451, index=3) -> (element=w447:dbl)
          n173 = for {
            tunnel: w444 -> [w462] mode=indexing
            tunnel: [w461] -> w442 mode=indexing
            tunnel: w440 -> [w460]
            n174 = Format Into String(format string=w462, w460) -> (resulting string=w461:string)  [unwired: 2 in, 1 out]
          }
          n175 = call "Number_2_string.vi"("number"=w450) -> ("String"=w458:string)  [unwired: 1 in]
          n176 = call "Number_2_string.vi"("number"=w449) -> ("String"=w459:string)  [unwired: 1 in]
          n177 = call "Number_2_string.vi"("number"=w448) -> ("String"=w457:string)  [unwired: 1 in]
          n178 = Number To Decimal String(number=w447) -> (decimal integer string=w456:string)  [unwired: 1 out]
          n179 = Build Array (concatenate)(w446, w458, w459, w457, w456) -> (w445:string[])
          n180 = Build Array (concatenate)(w443, w442) -> (w441:string[])
        }
        "Plug in titles" <- w416
        "Plug in values" <- w418
        n181 = Decimal String To Number(string=w399) -> (number=w396:i32[])  [unwired: 2 in, 1 out]
        n182 = Index Array(array=w398, index (col)=0 ("disabled index (col)")) -> (element=w395:dbl[])  [unwired: 1 in]
        n183 = local read "Laser Disp Index"() -> (w414:i32)
        n184 = Bundle(w396, "All WTs"=w395) -> (→"Turbine RPMs":cluster{i32[], "All WTs":dbl[]})  [unwired: 1 in]
        n185 = Greater Or Equal To 0?(x=w414) -> (x >= 0?=w413:bool)
        n186 = Select(t="Laser Displacement Analysis", s=w413, f="Get Last Block info") -> (s? t:f=w412:string)
      }
      frame "Laser Displacement Analysis" {
        # "L"
        # "S"
        # "R"
        # "D^2"
        # "D"
        n187 = stacked-sequence {
          seq-local: [_ w481 _ _ _ _ _] -> [_ _ w499 _ _ _ _]
          seq-local: [_ _ w500 _ _ _ _] -> [_ _ _ _ w566 _ _]
          seq-local: [w474 _ _ _ _ _ _] -> [_ _ _ _ w562 _ _]
          seq-local: [w475 _ _ _ _ _ _] -> [_ _ _ _ w561 _ _]
          seq-local: [_ _ _ w536 _ _ _] -> [_ _ _ _ w554 _ _]
          seq-local: [_ _ _ w531 _ _ _] -> [_ _ _ _ w553 _ _]
          seq-local: [_ _ _ w534 _ _ _] -> [_ _ _ _ w552 _ _]
          seq-local: [w475 _ _ _ _ _ _] -> [_ w482 _ _ _ _ _]
          tunnel: w473 -> [_ _ _ _ _ _ _]
          tunnel: w472 -> [_ _ _ _ _ _ _]
          tunnel: w471 -> [_ _ _ w532 w555 _ _]
          tunnel: w470 -> [_ _ _ _ _ w640 w678]
          tunnel: [_ _ _ _ _ TRUE _] -> w469
          tunnel: [_ _ _ _ _ "Get Last Block info" _] -> w468
          tunnel: w464 -> [w478 w485 _ _ _ _ _]
          tunnel: w463 -> [_ _ _ w550 _ _ _]
          frame #0 {
            n188 = local read "Laser Phase lock index"() -> (w476:i32)
            n189 = Index Array(array=w478, index=w476) -> (element=w477:cluster{dbl[], dbl[]})
            n190 = Unbundle(w477) -> (w475:dbl[], w474:dbl[])
            n191 = Build Array (concatenate)(w475, w475, 0.0) -> ()  [unwired: 1 out]
            n192 = Build Array (concatenate)(w474, w474, 0.0) -> ()  [unwired: 1 out]
          }
          frame #1 {
            n193 = local read "Laser Status Index"() -> (w484:i32)
            n194 = Less Than 0?(x=w484) -> (x < 0?=w483:bool)
            n195 = case shown="True" w483 {
              tunnel: w485 -> [w491 _]
              tunnel: w482 -> [_ w498]
              tunnel: [w487 w493] -> w481
              frame False {
                n196 = local read "L Status Phase lock index"() -> (w490:i32)
                n197 = Index Array(array=w491, index=w490) -> (element=w492:cluster{dbl[], dbl[]})
                n198 = Unbundle(w492) -> (w486:dbl[])  [unwired: 1 out]
                n199 = Build Array (concatenate)(w486, w486, 0.0) -> ()  [unwired: 1 out]
                n200 = Greater?(x=w486, y=0.4) -> (0:w487:bool[])
              }
              frame True {
                n201 = Greater?(x=w498, y=-5) -> (0:w494:bool[])
                n202 = Build Array (concatenate)(w494, w494, FALSE) -> (w495:bool[])
                n203 = Not(x=w495) -> (.not. x?=w493:bool[])
              }
            }
          }
          frame #2 {
            n204 = Index Array(array=w499, index=0) -> (element=w502:bool)
            n205 = for {
              tunnel: w499 -> [w509] mode=indexing
              shift-right: [w509] -> _
              shift-left: w502 -> [w504]
              shift-right: [w506] -> w500
              shift-left: i32[] [] -> [w507]
              i -> [w508]
              n206 = Not Equal?(x=w509, y=w504) -> (x != y?=w505:bool)
              n207 = case shown="True" w505 {
                tunnel: w508 -> [_ w516]
                tunnel: w507 -> [w510 w514]
                tunnel: [w510 w515] -> w506
                tunnel: w504 -> [_ w511]
                frame False {
                }
                frame True {
                  n208 = Array Size(array=w514) -> (size(s)=w513:i32)
                  n209 = Equal To 0?(x=w513) -> (x = 0?=w512:bool)
                  n210 = case shown="True" w512 {
                    tunnel: w516 -> [w517 w523]
                    tunnel: w514 -> [w519 w522]
                    tunnel: [w518 w521] -> w515
                    tunnel: w511 -> [_ w520]
                    frame False {
                      n211 = Build Array (concatenate)(w519, w517) -> (w518:i32[])
                    }
                    frame True {
                      n212 = case shown="False" w520 {
                        tunnel: w523 -> [_ w527]
                        tunnel: w522 -> [w524 w526]
                        tunnel: [w524 w525] -> w521
                        frame False {
                        }
                        frame True {
                          n213 = Build Array (concatenate)(w526, w527) -> (w525:i32[])
                        }
                      }
                    }
                  }
                }
              }
            }
          }
          frame #3 {
            n214 = local read "Laser Disp Index"() -> (w549:i32)
            n215 = Index Array(array=w550, index=w549) -> (element=w551:T2)
            n216 = Unbundle By Name(w551) -> ("Y"=w542:dbl)
            n217 = Absolute Value(x=w542) -> (abs(x)=w536:dbl)
            n218 = formula code="S=(0.0001*R*R) -0.0619*R+7.7094;"("R"=w536) -> ("S"=w530:dbl)
            n219 = Divide(x=10, y=w536) -> (x/y=w547:dbl)
            n220 = Inverse Tangent(1:w547) -> (0:w546:dbl)
            n221 = Divide(x=w546, y=3.141592653589793) -> (x/y=w544:dbl)
            n222 = Max & Min(x=w530, y=0.0) -> (max(x,y)=w528:dbl)  [unwired: 1 out]
            n223 = Divide(x=w528, y=w536) -> (x/y=w537:dbl)
            n224 = Inverse Tangent(1:w537) -> (0:w538:dbl)
            n225 = Divide(x=w538, y=3.141592653589793) -> (x/y=w540:dbl)
            n226 = Multiply(x=w544, y=180.0) -> (x*y=w533:dbl)
            n227 = Multiply(x=w540, y=180.0) -> (x*y=w535:dbl)
            n228 = Divide(x=w535, y=w532) -> (x/y=w534:dbl)
            n229 = Divide(x=w533, y=w532) -> (x/y=w531:dbl)
          }
          frame #4 {
            w556 = 360.0 ("y")
            n230 = Divide(x="Start Cut Deg", y=w555) -> (x/y=w568:dbl)
            n231 = Divide(x="End Cut Deg", y=w555) -> (x/y=w569:dbl)
            n232 = To Long Integer(number=w568) -> (32bit integer=w564:i32)
            n233 = To Long Integer(number=w569) -> (32bit integer=w567:i32)
            n234 = Add(x=w564, y=w567) -> (x+y=w563:i32)
            n235 = Divide(x=w555, y=w556) -> (x/y=w560:dbl)
            n236 = Multiply(x=w560, y=6.283185307179586) -> (x*y=w559:dbl)
            n237 = Multiply(x=w559, y=w554) -> (x*y=w557:dbl)
            n238 = for {
              N: 3 -> [_]
              tunnel: w561 -> [w607]
              tunnel: w566 -> [w604]
              tunnel: w564 -> [w574]
              tunnel: w563 -> [w600]
              tunnel: w557 -> [w599]
              tunnel: w562 -> [w591]
              tunnel: w556 -> [w584]
              tunnel: w555 -> [w578]
              tunnel: w553 -> [w576]
              tunnel: w552 -> [w572]
              i -> [w598]
              n239 = Multiply(x=w598, y=2) -> (x*y=w602:i32)
              n240 = Increment(x=w602) -> (x+1=w601:i32)
              n241 = Index Array(array=w604, index=w602) -> (element=w609:i32)
              n242 = Index Array(array=w604, index=w601) -> (element=w610:i32)
              n243 = Subtract(x=w610, y=w609) -> (x-y=w608:i32)
              n244 = Add(x=w572, y=w574) -> (x+y=w573:dbl)
              n245 = Add(x=w609, y=w573) -> (x+y=w594:dbl)
              n246 = Subtract(x=w608, y=w600) -> (x-y=w577:i32)
              n247 = Max & Min(x=w577, y=w576) -> (min(x,y)=w575:dbl)  [unwired: 1 out]
              n248 = Array Subset(array=w591, index=w594, length=w575) -> (w582:dbl[])
              n249 = call-poly <vilib>:"Mean.vi"("X"=w582) -> ("mean"=w581:dbl)  [unwired: 1 out]
              n250 = Multiply(x=2.0, y=w581) -> (x*y=w579:dbl)
              n251 = call "Top_and_Tail_ph.vi"("Array in"=w582, "Threshold"=w579) -> ("Length"=w589:i32, "Start Index"=w593:i32)
              n252 = Add(x=w594, y=w593) -> (x+y=w590:dbl)
              n253 = Array Subset(array=w591, index=w590, length=w589) -> (w592:dbl[])
              n254 = call-poly <vilib>:"Mean.vi"("X"=w592) -> ("mean"=w595:dbl)  [unwired: 1 out]
              n255 = Array Subset(array=w607, index=w590, length=w589) -> (w597:dbl[])
              n256 = Array Size(array=w597) -> (size(s)=w606:i32)
              n257 = for {
                N: w606 -> [_]
                tunnel: w599 -> [w637]
                tunnel: [w635] -> w605 mode=indexing
                i -> [w636]
                n258 = Multiply(x=w636, y=w637) -> (x*y=w635:dbl)
              }
              n259 = call <vilib>:"Linear Fit.vi"("Y"=w597, "X"=w605) -> ("slope"=w588:dbl)  [unwired: 9 in, 4 out]
              n260 = call-poly <vilib>:"Mean.vi"("X"=w597) -> ("mean"=w596:dbl)  [unwired: 1 out]
              n261 = Inverse Tangent(1:w588) -> (0:w587:dbl)
              n262 = Divide(x=w587, y=6.283185307179586) -> (x/y=w585:dbl)
              n263 = Multiply(x=w585, y=w584) -> (x*y=w583:dbl)
              n264 = case shown="2" w598 {
                tunnel: w597 -> [w614 w621 w628]
                tunnel: w588 -> [w618 w625 w633]
                tunnel: w596 -> [w617 w626 w634]
                tunnel: w592 -> [_ _ _]
                tunnel: w595 -> [w616 w624 w632]
                tunnel: w583 -> [w615 w623 w631]
                tunnel: w578 -> [w611 w622 w629]
                frame 0, Default {
                  n265 = Bundle(0.0, "Angular Step"=w611, w614) -> (→"Mean Blade 1":cluster{dbl, "Angular Step":dbl, dbl[]})  [unwired: 1 in]
                  "slope 1" <- w618
                  "Av Disp 1" <- w617
                  "Av Variance 1" <- w616
                  "Angle 1" <- w615
                }
                frame 1 {
                  n266 = Bundle(0.0, "Angular Step"=w622, w621) -> (→"Mean Blade 2":cluster{dbl, "Angular Step":dbl, dbl[]})  [unwired: 1 in]
                  "Av Disp 2" <- w626
                  "slope 2" <- w625
                  "Av Variance 2" <- w624
                  "Angle 2" <- w623
                }
                frame 2 {
                  n267 = Bundle(0.0, "Angular Step"=w629, w628) -> (→"Mean Blade 3":cluster{dbl, "Angular Step":dbl, dbl[]})  [unwired: 1 in]
                  "Av Disp 3" <- w634
                  "slope 3" <- w633
                  "Av Variance 3" <- w632
                  "Angle 3" <- w631
                }
              }
            }
          }
          frame #5 {
            n268 = case shown="True" w640 {
              frame False {
              }
              frame True {
                n269 = for {
                  N: 3 -> [_]
                  tunnel: [w671] -> w662 mode=indexing
                  tunnel: [w670] -> w661 mode=indexing
                  tunnel: [w669] -> w660 mode=indexing
                  tunnel: [w668] -> w644 mode=indexing
                  i -> [w677]
                  n270 = Increment(x=w677) -> (x+1=w676:i32)
                  n271 = Format Into String(format string="Blade %d:", w676) -> (resulting string=w667:string)  [unwired: 2 in, 1 out]
                  n272 = Concatenate Strings(w667, "Angle:") -> (w668:string)
                  n273 = Concatenate Strings(w667, "Slope:") -> (w671:string)
                  n274 = Concatenate Strings(w667, "Average:X") -> (w670:string)
                  n275 = Concatenate Strings(w667, "Variance of:X") -> (w669:string)
                }
                n276 = local read "Av Variance 1"() -> (w651:dbl)
                n277 = local read "Av Variance 2"() -> (w650:dbl)
                n278 = local read "Av Variance 3"() -> (w649:dbl)
                n279 = local read "Av Disp 1"() -> (w654:dbl)
                n280 = local read "Av Disp 2"() -> (w653:dbl)
                n281 = local read "Av Disp 3"() -> (w652:dbl)
                n282 = local read "slope 1"() -> (w657:dbl)
                n283 = local read "slope 2"() -> (w656:dbl)
                n284 = local read "slope 3"() -> (w655:dbl)
                n285 = local read "Angle 3"() -> (w643:dbl)
                n286 = local read "Angle 1"() -> (w642:dbl)
                n287 = local read "Angle 2"() -> (w641:dbl)
                n288 = Build Array(w642, w641, w643, w657, w656, w655, w654, w653, w652, w651, w650, w649) -> (w648:dbl[])
                n289 = local read "Plug in values"() -> (w647:string[])
                n290 = local read "Plug in titles"() -> (w659:string[])
                n291 = for {
                  tunnel: w648 -> [w665] mode=indexing
                  tunnel: [w664] -> w646 mode=indexing
                  n292 = call "Number_2_string.vi"("number"=w665) -> ("String"=w664:string)  [unwired: 1 in]
                }
                n293 = Build Array (concatenate)(w659, w644, w662, w661, w660) -> (w658:string[])
                n294 = Build Array (concatenate)(w647, w646) -> (w645:string[])
                n295 = local write "Plug in titles"(w658) -> ()
                n296 = local write "Plug in values"(w645) -> ()
              }
            }
          }
          frame #6 {
            n297 = case shown="True" w678 {
              frame False {
              }
              frame True {
                n298 = local read "Blade Analysis"() -> (w682:string[][])
                n299 = for {
                  tunnel: [w687] -> w685 mode=concatenating
                  tunnel: w682 -> [w686] mode=indexing
                  tunnel: [w686] -> w679 mode=concatenating
                  i -> [w699]
                  n300 = Increment(x=w699) -> (x+1=w698:i32)
                  n301 = Format Into String(format string="Blade %d:", w698) -> (resulting string=w693:string)  [unwired: 2 in, 1 out]
                  n302 = Concatenate Strings(w693, "Angle:Degrees") -> (w691:string)
                  n303 = Concatenate Strings(w693, "Angle:Variance") -> (w690:string)
                  n304 = Concatenate Strings(w693, "Position:(mm)") -> (w689:string)
                  n305 = Concatenate Strings(w693, "Position:Variance") -> (w688:string)
                  n306 = Build Array(w691, w690, w689, w688) -> (w687:string[])
                }
                n307 = local read "Plug in titles"() -> (w684:string[])
                n308 = local read "Plug in values"() -> (w681:string[])
                n309 = Build Array (concatenate)(w684, w685) -> (w683:string[])
                n310 = Build Array (concatenate)(w681, w679) -> (w680:string[])
                n311 = local write "Plug in values"(w680) -> ()
                n312 = local write "Plug in titles"(w683) -> ()
              }
            }
          }
        }
      }
      frame "Get Last Block info" {
        n313 = case shown="\"Take New Data\"" w707 {
          tunnel: [w708 "Post Process"] -> w706
          tunnel: [w712 TRUE ("Processing last block?")] -> w705
          tunnel: w704 -> [w712 _]
          frame "Take New Data" {
            n314 = Select(t="Change Dem Volts", s="Change Dem Voltages?", f="Post Process") -> (s? t:f=w708:string)
          }
          frame "Post Process Raw Data File" {
          }
        }
      }
      frame "Change Dem Volts" {
        n315 = local read "WT Numbers"() -> (w717:string[])
        n316 = local read "All WTs"() -> (w743:dbl[][])
        n317 = for {
          N: 11 -> [_]
          tunnel: w747 -> [w773]
          tunnel: [w772] -> w746 mode=indexing
          tunnel: [w771] -> w729 mode=indexing
          tunnel: w743 -> [w769] mode=indexing
          tunnel: [w768] -> w741 mode=indexing
          tunnel: [w767] -> w723
          tunnel: w722 -> [w766]
          tunnel: w717 -> [w765] mode=indexing
          i -> [w774]
          n318 = Increment(x=w774) -> (x+1=w767:i32)
          n319 = Format Into String(format string=w773, w765) -> (resulting string=w771:string)  [unwired: 2 in, 1 out]
          n320 = Format Into String(format string=w766, w765) -> (resulting string=w772:string)  [unwired: 2 in, 1 out]
          n321 = Index Array(array=w769, index=0) -> (element=w768:dbl)
        }
        n322 = Build Array (concatenate)(w746, w729) -> (w745:string[])
        n323 = call "Get_Current_Scan_client.vi"("ADAM Ch Names"=w745) -> ("Numerical Values"=w744:dbl[])  [unwired: 3 out]
        n324 = Split 1D Array(array=w744, index=w723) -> (first subarray=w742:dbl[], second subarray=w740:dbl[])
        n325 = Divide(x=w742, y=w741) -> (x/y=w732:dbl[])
        n326 = In Range and Coerce(upper limit=1.05, x=w732, lower limit=0.95) -> (coerced(x)=w731:dbl[], In Range?=w730:bool[])
        n327 = Multiply(x=w731, y=w740) -> (x*y=w735:dbl[])
        n328 = In Range and Coerce(upper limit=9.9, x=w735, lower limit=0.0) -> (coerced(x)=w728:dbl[])  [unwired: 1 out]
        n329 = for {
          shift-right: [w755] -> w726
          shift-left: string[] [] -> [w756]
          shift-right: [w753] -> w727
          shift-left: dbl[] [] -> [w754]
          tunnel: w730 -> [w750] mode=indexing
          tunnel: w729 -> [w752] mode=indexing
          tunnel: w728 -> [w751] mode=indexing
          tunnel: "Allow large changes?" -> [w748]
          n330 = Or(x=w748, y=w750) -> (x .or. y?=w749:bool)
          n331 = case shown="False" w749 {
            tunnel: w756 -> [w758 w764]
            tunnel: [w758 w763] -> w755
            tunnel: w754 -> [w757 w762]
            tunnel: [w757 w761] -> w753
            tunnel: w752 -> [_ w760]
            tunnel: w751 -> [_ w759]
            frame False {
            }
            frame True {
              n332 = Build Array (concatenate)(w764, w760) -> (w763:string[])
              n333 = Build Array (concatenate)(w762, w759) -> (w761:dbl[])
            }
          }
        }
        n334 = call "ASYNC_Adam_client.vi"("Values"=w727, "Channel Names"=w726) -> ()  [unwired: 2 out]
      }
      frame "Post Process" {
        n335 = Compound Arithmetic op=AND("Add Phase data to results file", w781) -> (w780:bool)
        n336 = case shown="True" w780 {
          tunnel: w779 -> [_ w787]
          tunnel: w775 -> [_ w786]
          frame False {
          }
          frame True {
            n337 = stacked-sequence {
              tunnel: w787 -> [w789 _]
              tunnel: w786 -> [_ w815]
              frame #0 {
                n338 = local read "Channel to Phase lock"() -> (w796:i32[])
                n339 = property on="Channel to Phase lock" class="LstBox (strict)"() -> ("Item Names"=w795:string[])  [unwired: 2 in, 2 out]
                n340 = local read "Plug in titles"() -> (w790:string[])
                n341 = Divide(x=360, y=w789) -> (x/y=w792:dbl)
                n342 = Increment(x=w789) -> (x+1=w788:dbl)
                n343 = for {
                  tunnel: w795 -> [w814]
                  tunnel: w796 -> [w813] mode=indexing
                  tunnel: [w812] -> w794 mode=indexing
                  n344 = Index Array(array=w814, index=w813) -> (element=w812:string)
                }
                n345 = for {
                  tunnel: w794 -> [w803] mode=indexing
                  tunnel: w792 -> [w802]
                  shift-right: [w799] -> w791
                  shift-left: w790 -> [w801]
                  tunnel: w788 -> [w797]
                  n346 = for {
                    N: w797 -> [_]
                    tunnel: w803 -> [w806]
                    tunnel: w802 -> [w810]
                    tunnel: [w808] -> w800 mode=indexing
                    tunnel: [w805] -> w798 mode=indexing
                    i -> [w811]
                    n347 = Multiply(x=w810, y=w811) -> (x*y=w804:dbl)
                    n348 = Format Into String(format string="%s:Mean:%.1f Deg:%.1f", w806, w804, w804) -> (resulting string=w808:string)  [unwired: 2 in, 1 out]
                    n349 = Format Into String(format string="%s:Variance:%.1f Deg:%.1f", w806, w804, w804) -> (resulting string=w805:string)  [unwired: 2 in, 1 out]
                  }
                  n350 = Build Array (concatenate)(w801, w800, w798) -> (w799:string[])
                }
                n351 = local write "Plug in titles"(w791) -> ()
              }
              frame #1 {
                n352 = local read "Plug in values"() -> (w817:string[])
                n353 = for {
                  tunnel: w815 -> [w820] mode=indexing
                  shift-right: [w823] -> w816
                  shift-left: w817 -> [w824]
                  n354 = Unbundle(w820) -> (w818:dbl[], w819:dbl[])
                  n355 = for {
                    tunnel: w818 -> [w827] mode=indexing
                    tunnel: [w828] -> w822 mode=indexing
                    tunnel: w819 -> [w825] mode=indexing
                    tunnel: [w826] -> w821 mode=indexing
                    n356 = call "Number_2_string.vi"("number"=w827) -> ("String"=w828:string)  [unwired: 1 in]
                    n357 = call "Number_2_string.vi"("number"=w825) -> ("String"=w826:string)  [unwired: 1 in]
                  }
                  n358 = Build Array (concatenate)(w824, w822, w821) -> (w823:string[])
                }
                n359 = local write "Plug in values"(w816) -> ()
              }
            }
          }
        }
        n360 = Compound Arithmetic op=AND("Save Phase averaged Profiles", w781) -> (w783:bool)
      }
      frame "Check Folder Name" {
        n361 = File/Directory Info(path="Output Directory") -> (error out=w837:errorcluster)  [unwired: 1 in, 6 out]
        n362 = Empty String/Path?(string/path="Output Directory") -> (empty?=w839:bool)
        n363 = Unbundle By Name(w837) -> ("status"=w838:bool)
        n364 = Or(x=w839, y=w838) -> (x .or. y?=w840:bool)
        n365 = case shown="True" w840 {
          tunnel: [w843 w849] -> w833
          tunnel: "Output Directory" -> [w843 w847]
          tunnel: [FALSE ("cancelled") w844] -> w835
          frame False {
          }
          frame True {
            n366 = Strip Path(path=w847) -> (stripped path=w846:path, name=w845:string)
            n367 = File Dialog(7:"Please Select a new or existing Results folder" ("prompt"), 9:w845, 11:w846) -> (1:w844:bool, 3:w849:path)  [unwired: 1 in, 5 out]
          }
        }
        n368 = local write "Output Directory"(w833) -> ()
        n369 = Not(x=w835) -> (.not. x?=w834:bool)
      }
      frame "Save Phase locked data" {
        n370 = global read "Meas_global.vi" "Raw data file"() -> (w856:path)
        n371 = stacked-sequence {
          seq-local: [_ w886 _ _] -> [_ _ _ w944]
          seq-local: [w864 _ _ _] -> [_ _ _ w945]
          seq-local: [_ _ w901 _] -> [_ _ _ w943]
          seq-local: [w859 _ _ _] -> [_ _ w900 _]
          tunnel: w857 -> [_ _ _ _]
          tunnel: w856 -> [w863 _ _ w949]
          tunnel: w852 -> [w862 _ _ _]
          tunnel: w851 -> [_ _ w899 _]
          frame #0 {
            w865 = "\r\n"
            n372 = for {
              tunnel: w862 -> [w870] mode=indexing
              tunnel: [w868] -> w861 mode=indexing
              tunnel: [w869] -> w860 mode=indexing
              n373 = Unbundle(w870) -> (w868:dbl[], w869:dbl[])
            }
            n374 = call "Read_RD_Ch_header.vi"("Raw data file"=w863) -> ("Ch string"=w867:string)  [unwired: 3 out]
            n375 = Concatenate Strings(w865, "*****This is a many rows per single point file*****", w865, w867) -> (w864:string)
            n376 = Build Array (concatenate)(w861, w860) -> (w859:dbl[][])
          }
          frame #1 {
            w872 = "\r\n"
            n377 = local read "Channel to Phase lock"() -> (w888:i32[])
            n378 = property on="Channel to Phase lock" class="LstBox (strict)"() -> ("Item Names"=w887:string[])  [unwired: 2 in, 2 out]
            n379 = Initialize Array("", 10) -> (w889:string[])
            n380 = call "Asterisk_header.vi"("Channel names"=w889) -> ("Header string"=w871:string)
            n381 = for {
              tunnel: w888 -> [w897] mode=indexing
              tunnel: w887 -> [w896]
              tunnel: [w895] -> w884 mode=indexing
              tunnel: ["Mean" ("format string")] -> w882 mode=indexing
              tunnel: ["Variance" ("format string")] -> w881 mode=indexing
              tunnel: [""] -> w879 mode=indexing
              n382 = Index Array(array=w896, index=w897) -> (element=w895:string)
            }
            n383 = Build Array (concatenate)("Rotor", w884, w884) -> (w878:string[])
            n384 = Build Array (concatenate)("Angle", w882, w881) -> (w877:string[])
            n385 = Build Array (concatenate)("(deg)", w879, w879) -> (w876:string[])
            n386 = Build Array(w878, w877, w876) -> (w875:string[][])
            n387 = Array To Spreadsheet String(array=w875, 3:"%s" ("format string")) -> (spreadsheet string=w873:string)  [unwired: 1 out]
            n388 = Concatenate Strings(w872, w871, w873, w872) -> (w886:string)
          }
          frame #2 {
            n389 = Array Size(array=w900) -> (size(s)=w902:i32[])
            n390 = Index Array(array=w902, index=0) -> (element=w907:i32)
            n391 = Index Array(array=w902, index=1) -> (element=w903:i32)
            n392 = Decrement(x=w907) -> (x-1=w908:i32)
            n393 = for {
              N: w903 -> [_]
              shift-right: [w924] -> w901
              shift-left: "" -> [w919]
              tunnel: "Separation Character" -> [w916]
              tunnel: w900 -> [w922]
              tunnel: w908 -> [w918]
              tunnel: w899 -> [w913]
              tunnel: [w909] -> _ mode=indexing
              i -> [w915]
              n394 = Divide(x=w913, y=2.0) -> (x/y=w911:dbl)
              n395 = Multiply(x=w915, y=w913) -> (x*y=w910:dbl)
              n396 = Index Array(array=w922, index (col)=w915) -> (element=w921:dbl[])  [unwired: 1 in]
              n397 = Add(x=w910, y=w911) -> (x+y=w909:dbl)
              n398 = call "Number_2_string.vi"("number"=w909) -> ("String"=w914:string)  [unwired: 1 in]
              n399 = Concatenate Strings(w914, w916) -> (w917:string)
              n400 = for {
                shift-right: [w932] -> w920
                shift-left: w917 -> [w933]
                tunnel: w916 -> [w931]
                tunnel: w921 -> [w927] mode=indexing
                tunnel: w918 -> [w929]
                i -> [w930]
                n401 = Equal?(x=w930, y=w929) -> (x = y?=w928:bool)
                n402 = call "Number_2_string.vi"("precision"="precision", "number"=w927) -> ("String"=w926:string)
                n403 = case shown="False" w928 {
                  tunnel: w933 -> [w937 w940]
                  tunnel: w926 -> [w936 w939]
                  tunnel: [w935 w938] -> w932
                  tunnel: w931 -> [w934 _]
                  frame False {
                    n404 = Concatenate Strings(w937, w936, w934) -> (w935:string)
                  }
                  frame True {
                    n405 = Concatenate Strings(w940, w939) -> (w938:string)
                  }
                }
              }
              n406 = Concatenate Strings(w919, w920, "\r\n") -> (w924:string)
            }
          }
          frame #3 {
            w941 = FALSE  # append to file? (new file:F)
            n407 = Strip Path(path=w949) -> (name=w947:string)  [unwired: 1 out]
            n408 = local read "Output Directory"() -> (w948:path)
            n409 = Build Path(base path=w948, name or relative path=w947) -> (appended path=w946:path)
            n410 = Concatenate Strings(w945, w944, w943) -> (w942:string)
            n411 = call "Write_File_Simple.vi"("append to file? (new file:F)"=w941, "character string"=w942, "file path"=w946) -> ()  [unwired: 2 out]
          }
        }
      }
    }
  }
